vi "demo.vi"() -> ()   [LabVIEW 2013]
panel:
  in  "取消注册":bool
  out "采集数据":dbl[][](array[numeric])
  in  "停止":bool
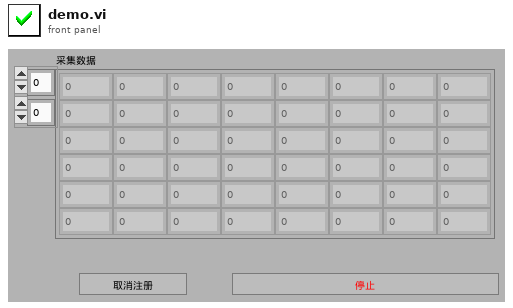
[diagram p1: front panel]
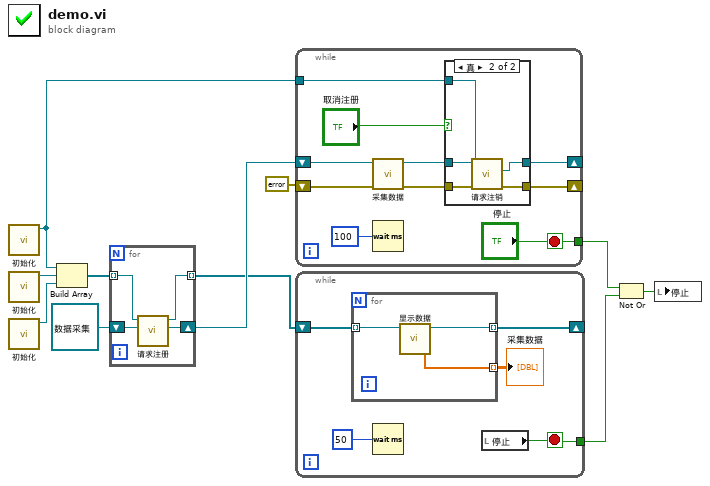
[diagram p0: block diagram]
diagram:
  n1 = call "初始化.vi"() -> ("数据存储 输出"=w4:refnum<class "数据存储.lvclass">)  [unwired: 9 in, 1 out]
  n2 = call "初始化.vi"() -> ("数据分析 输出"=w10:refnum<class "数据分析.lvclass">)  [unwired: 9 in, 1 out]
  n3 = call "初始化.vi"() -> ("数据显示 输出"=w9:refnum<class "数据显示.lvclass">)  [unwired: 9 in, 1 out]
  n4 = Build Array(w4, w10, w9) -> (w7:refnum<class "订阅者接口.lvclass">[])
  n5 = for {
    shift-right: [w13] -> w6
    shift-left: refnum<class "数据采集.lvclass"> refnum ("数据采集.lvclass") -> [w14]
    tunnel: w7 -> [w15] mode=indexing
    tunnel: [w12] -> w5 mode=indexing
    n6 = call-dynamic "请求注册.vi"("数据采集.lvclass"=w14, "订阅者接口 输入"=w15) -> ("数据采集.lvclass"=w13:refnum<class "数据采集.lvclass">, "订阅者接口 输出"=w12:refnum<class "订阅者接口.lvclass">)  [unwired: 7 in, 1 out]
  }
  n7 = while {
    shift-right: [w19] -> _
    shift-left: w6 -> [w24]
    shift-right: [w21] -> _
    shift-left: errorcluster {"status"=FALSE, "code"=0, "source"=""} ("error out") -> [w23]
    tunnel: w4 -> [w17]
    tunnel: ["停止"] -> w3
    stop <- "停止" stop-if-true
    n8 = call "采集数据.vi"("error in (no error)"=w23, "数据采集 输入"=w24) -> ("error out"=w22:errorcluster, "数据采集 输出"=w20:refnum<class "数据采集.lvclass">)  [unwired: 8 in]
    n9 = Wait (ms)(milliseconds to wait=u32 100 ("等待时间（毫秒）")) -> ()  [unwired: 1 out]
    n10 = case shown="真" "取消注册" {
      tunnel: w22 -> [w26 w29]
      tunnel: [w26 w28] -> w21
      tunnel: w20 -> [w27 w31]
      tunnel: [w27 w30] -> w19
      tunnel: w17 -> [_ w32]
      frame False {
      }
      frame True {
        n11 = call-dynamic "请求注销.vi"("error in (no error)"=w29, "数据采集.lvclass"=w31, "数据存储 输入"=w32) -> ("error out"=w28:errorcluster, "数据采集.lvclass"=w30:refnum<class "数据采集.lvclass">)  [unwired: 6 in, 1 out]
      }
    }
  }
  n12 = while {
    shift-right: [w35] -> _
    shift-left: w5 -> [w36]
    tunnel: [w33] -> w2
    stop <- w33 stop-if-true
    n13 = for {
      tunnel: w36 -> [w40] mode=indexing
      tunnel: [w39] -> w35 mode=indexing
      tunnel: [w38] -> w34 mode=indexing
      n14 = call-dynamic "显示数据.vi"("订阅者接口 输入"=w40) -> ("采集数据"=w38:dbl[], "订阅者接口 输出"=w39:refnum<class "订阅者接口.lvclass">)  [unwired: 8 in, 1 out]
    }
    "采集数据" <- w34
    n15 = Wait (ms)(milliseconds to wait=u32 50 ("等待时间（毫秒）")) -> ()  [unwired: 1 out]
    n16 = local read "停止"() -> (w33:bool)
  }
  n17 = Not Or(1:w2, 2:w3) -> (0:w1:bool)
  n18 = local write "停止"(w1) -> ()
